vi "Set Channel Values.vi"(8 "error in (no error)":errorcluster, 10 "Alias Value Pairs in":cluster{"Alias":string, "Value":dbl}[](array[cluster]), 11 "SLSC EDS System Tests in":refnum<class "SLSC EDS System Tests.lvclass">) -> (0 "error out":errorcluster, 3 "SLSC EDS System Tests out":refnum<class "SLSC EDS System Tests.lvclass">)   [LabVIEW 2015, in "SLSC EDS System Tests.lvclass"]
uses:
  SLSC EDS System Tests.lvclass
  <vilib>/NI Veristand/Execution/Workspace/NI VeriStand - Set Multiple Channel Values.vi
  <vilib>/NI VeriStand/Execution/Workspace/NI_VS Workspace ExecutionAPI.lvlib
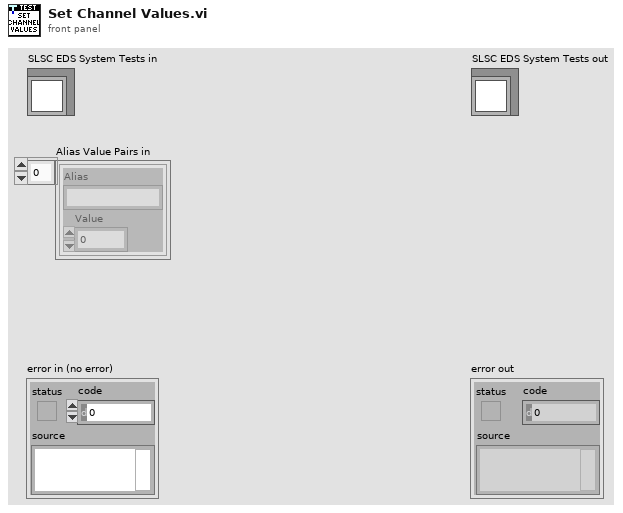
[diagram p1: front panel]
types:
  T1 = typedef "NI_VS Workspace ExecutionAPI.lvlib/WorkspaceAPI.ctl" = refnum<k24>
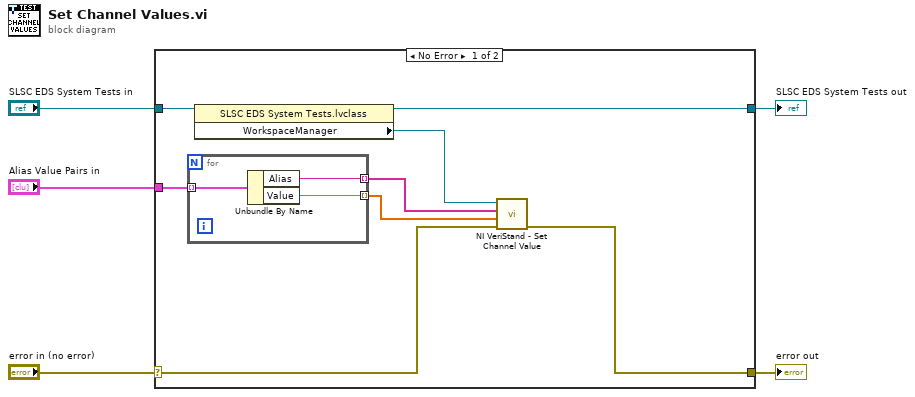
[diagram p0: block diagram]
diagram:
  n1 = case shown="No Error" "error in (no error)" {
    selector: "error in (no error)" -> [w13 w18]
    tunnel: [w12 w18] -> w4
    tunnel: [w9 w17] -> w2
    tunnel: "SLSC EDS System Tests in" -> [w10 w17]
    tunnel: "Alias Value Pairs in" -> [w8 _]
    frame No Error {
      n2 = for {
        tunnel: w8 -> [w16] mode=indexing
        tunnel: [w15] -> w7 mode=indexing
        tunnel: [w14] -> w6 mode=indexing
        n3 = Unbundle By Name(w16) -> ("Alias"=w15:string, "Value"=w14:dbl)
      }
      n4 = property class="SLSC EDS System Tests.lvclass"(reference=w10) -> (reference out=w9:refnum<class "SLSC EDS System Tests.lvclass">, "WorkspaceManager"=w11:T1)  [unwired: 1 in, 1 out]
      n5 = call-poly <vilib>:"NI VeriStand - Set Channel Value.vi"("error in (no error)"=w13, "Values"=w6, "Channels"=w7, "WorkspaceManager in"=w11) -> ("error out"=w12:errorcluster)  [unwired: 6 in, 1 out]
    }
    frame Error {
    }
  }
  "error out" <- w4
  "SLSC EDS System Tests out" <- w2
